vi "Labview file.vi"() -> ()   [LabVIEW 2017]
uses:
  <vilib>/Instr/_visa.llb/VISA Configure Serial Port (Instr).vi
panel:
  out "SPO2":dbl(graph)
  out "SPO2":dbl
  out "SPO2":dbl(knob) scale=0.0..200.0
  in  "INPUT USB":refnum<visa-resource-name>="COM13"
  out "Bytes Read":u32
  out "POS":dbl
  out "HEART":dbl
  out "POS":dbl(graph)
  out "HEART":dbl(graph)=4.0
  out "HEART":dbl(knob) scale=0.0..120.0
  out "POS":dbl(knob) scale=0.0..150.0
  in  "stop":bool
  # "Human Health Monitoring System"
  # "HEARTBEAT"
  # "POS"
  # "SP02"
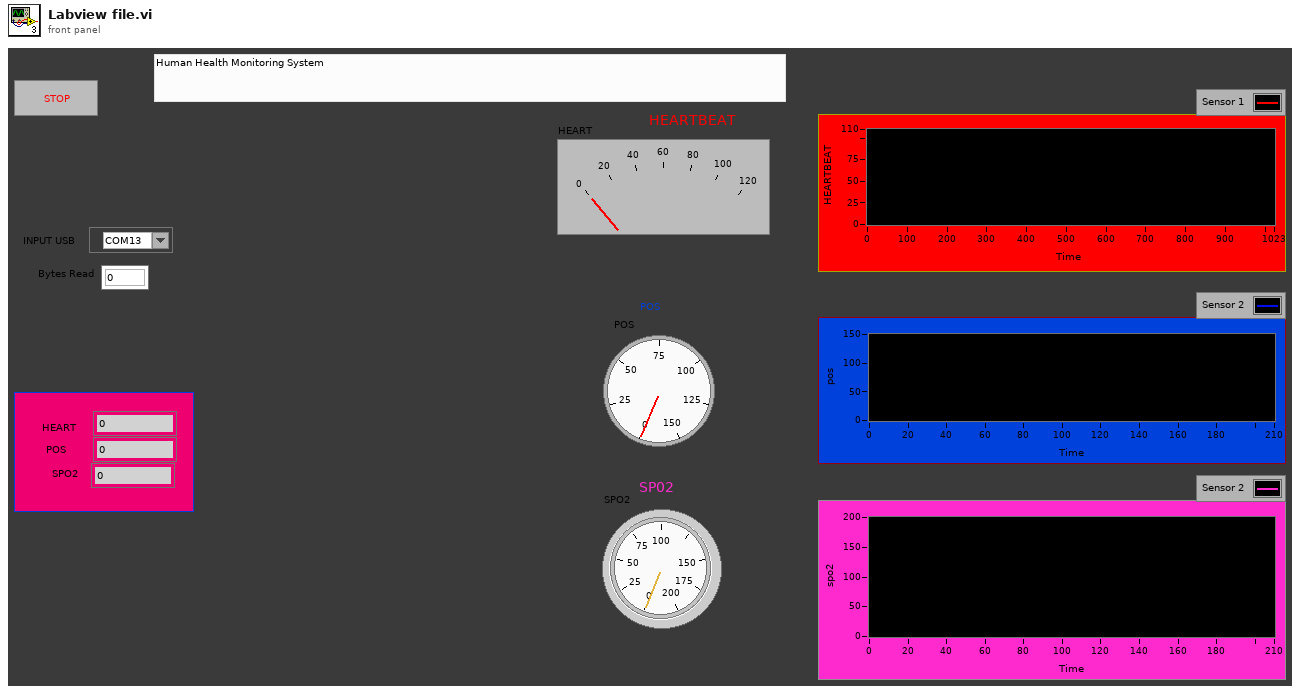
[diagram p1: front panel]
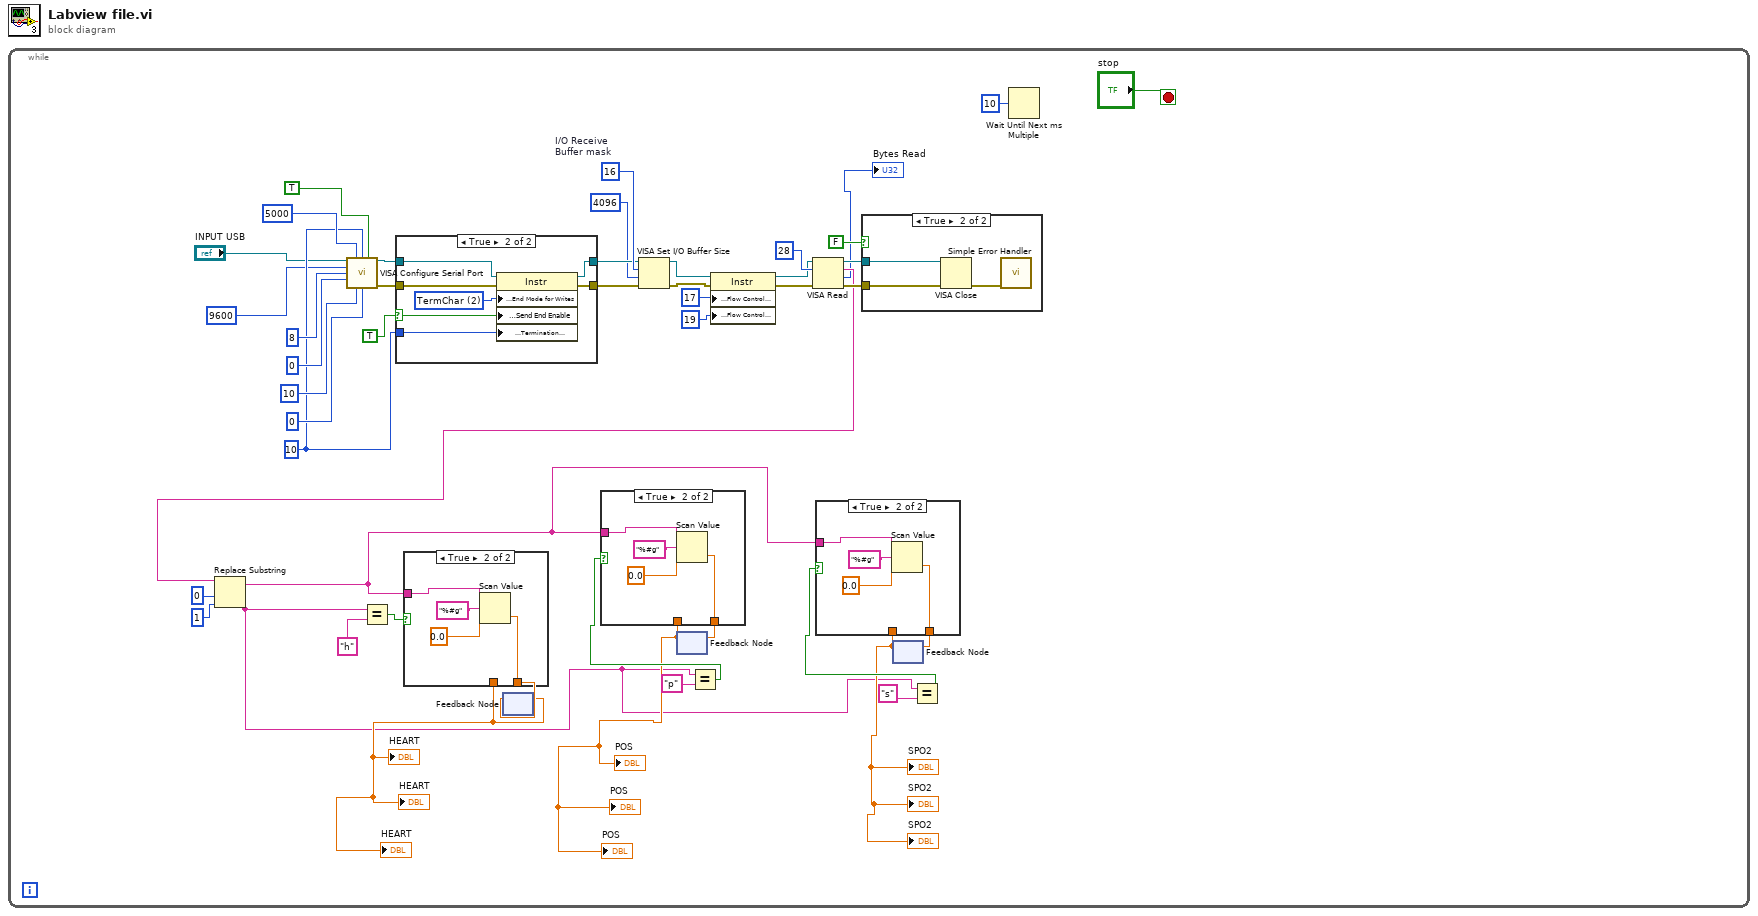
[diagram p0: block diagram]
diagram:
  n1 = while {
    stop <- "stop" stop-if-true
    w19 = u8 10
    w36 = u16 16  # I/O Receive Buffer mask
    n2 = call-poly "VISA Configure Serial Port"("VISA resource name"="INPUT USB", "timeout (10sec)"=u32 5000, "termination char\n(0xA = '\\n' = LF)"=w19, "Enable Termination\nChar (T)"=TRUE, "baud rate (9600)"=u32 9600, "data bits (8)"=u16 8, "parity (0:none)"=u16 0, "stop bits (10: 1 bit)"=u16 10, "flow control (0:none)"=u16 0) -> ("VISA resource name out"=w30:refnum<visa-resource-name>, "error out"=w33:errorcluster)  [unwired: 1 in, 4 out]
    n3 = case shown="True" TRUE {
      selector: TRUE -> [_ w57]
      tunnel: w30 -> [w55 w63]
      tunnel: w33 -> [w56 w62]
      tunnel: [w55 w61] -> w31
      tunnel: [w56 w60] -> w32
      tunnel: w19 -> [_ w58]
      frame False {
      }
      frame True {
        w59 = u16 2 items=["None", "LastBit", "TermChar", "Break"] ("Serial Settings:Serial End Mode for Writes")
        n4 = property class="Instr"(reference=w63, error in=w62, "Serial Settings:End Mode for Writes"=w59, "Message Based Settings:Send End Enable"=w57, "Message Based Settings:Termination Character"=w58) -> (reference out=w61:refnum<visa-resource-name>, error out=w60:errorcluster)
      }
    }
    n5 = feedback #1() -> (w10:dbl)  [unwired: 1 in]
    "HEART" <- w10
    "HEART" <- w10
    "HEART" <- w10
    n6 = VISA Set I/O Buffer Size(VISA resource name=w31, mask (16)=w36, size (4096)=u32 4096, error in (no error)=w32) -> (VISA resource name out=w35:refnum<visa-resource-name>, error out=w34:errorcluster)
    n7 = feedback #2() -> (w9:dbl)  [unwired: 1 in]
    "POS" <- w9
    "POS" <- w9
    "POS" <- w9
    n8 = property class="Instr"(reference=w35, error in=w34, "Serial Settings:Flow Control XON Character"=u8 17, "Serial Settings:Flow Control XOFF Character"=u8 19) -> (reference out=w13:refnum<visa-resource-name>, error out=w16:errorcluster)
    n9 = VISA Read(VISA resource name=w13, byte count=u32 28, error in (no error)=w16) -> (VISA resource name out=w15:refnum<visa-resource-name>, read buffer=w12:string, return count=→"Bytes Read":u32, error out=w14:errorcluster)
    n10 = Replace Substring(2:u8 1, 3:u8 0, 5:w12) -> (0:w1:string, 1:w2:string)  [unwired: 1 in]
    n11 = Equal?(x=w1, y="h") -> (x = y?=w43:bool)
    n12 = case shown="True" w43 {
      tunnel: w2 -> [_ w71]
      tunnel: [w69 w70] -> w41
      tunnel: w10 -> [w69 _]
      frame False {
      }
      frame True {
        n13 = Scan Value(string=w71, format string="%#g", default (0 dbl)=0.0) -> (value=w70:dbl)  [unwired: 1 out]
      }
    }
    n14 = feedback-in #1(w41) -> ()
    n15 = Equal?(x=w1, y="p") -> (x = y?=w40:bool)
    n16 = case shown="True" w40 {
      tunnel: w2 -> [_ w65]
      tunnel: [w64 w66] -> w39
      tunnel: w9 -> [w64 _]
      frame False {
      }
      frame True {
        n17 = Scan Value(string=w65, format string="%#g", default (0 dbl)=0.0) -> (value=w66:dbl)  [unwired: 1 out]
      }
    }
    n18 = feedback-in #2(w39) -> ()
    n19 = case shown="True" FALSE {
      tunnel: w15 -> [_ w53]
      tunnel: w14 -> [_ w52]
      frame False {
      }
      frame True {
        n20 = VISA Close(VISA resource name=w53, error in (no error)=w52) -> (error out=w54:errorcluster)
        n21 = call <vilib>:"Simple Error Handler.vi"("error in (no error)"=w54) -> ()  [unwired: 1 in, 8 out]
      }
    }
    n22 = feedback #3() -> (w3:dbl)  [unwired: 1 in]
    "SPO2" <- w3
    "SPO2" <- w3
    "SPO2" <- w3
    n23 = Equal?(x=w1, y="s") -> (x = y?=w5:bool)
    n24 = case shown="True" w5 {
      tunnel: w2 -> [_ w48]
      tunnel: [w47 w49] -> w4
      tunnel: w3 -> [w47 _]
      frame False {
      }
      frame True {
        n25 = Scan Value(string=w48, format string="%#g", default (0 dbl)=0.0) -> (value=w49:dbl)  [unwired: 1 out]
      }
    }
    n26 = feedback-in #3(w4) -> ()
    n27 = Wait Until Next ms Multiple(millisecond multiple=u32 10) -> ()  [unwired: 1 out]
  }
